vi "Create Debug Tool.vi"() -> (3 "array":T1)   [LabVIEW 2025, in "MCP Server.lvlib"]
uses:
  MCP Server.lvlib
  Tool Data.ctl
  Input Parameter.ctl
  Output Parameter.ctl
  Test_Tool.vi
  <vilib>/Utility/Data Type/NI_Data Type.lvlib
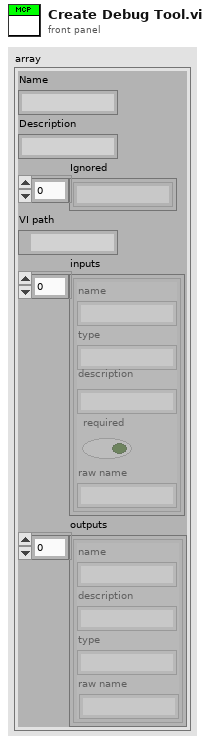
[diagram p1: front panel]
types:
  T1 = typedef "MCP Server.lvlib/Tool Data.ctl" = cluster{"Name":string, "Description":string, "Ignored":string[], "VI path":path, "inputs":T2[], "outputs":T3[]}
  T2 = typedef "MCP Server.lvlib/Input Parameter.ctl" = cluster{"name":string, "type":string, "description":string, "required":bool, "raw name":string}
  T3 = typedef "MCP Server.lvlib/Output Parameter.ctl" = cluster{"name":string, "description":string, "type":string, "raw name":string}
  T4 = enum16{"Invalid Wire Rule", "Required", "Recommended", "Optional", "Dynamic Dispatch"}[]
  T5 = enum16{"Invalid Wire Rule", "Required", "Recommended", "Optional", "Dynamic Dispatch"}
  T6 = typedef "NI_Data Type.lvlib/Data Type.ctl" = enum8{"Invalid Type", "Void", "I8", "I16", "I32", "I64", "U8", "U16", "U32", "U64", "Single Float", "Double Float", "Extended Float", "Single Complex", "Double Complex", "Extended Complex", "Enum U8", "Enum U16", "Enum U32", "Enum U64", "Single Float With Unit", "Double Float With Unit", "Extended Float With Unit", "Single Complex with Unit", "Double Complex with Unit", "Extended Complex with Unit", "Boolean", "String", "Path", "Picture", "Tag", "Array", "Cluster", "Variant", "LV Variant", "Waveform", "Timestamp", "Digital Waveform", "Digital Data", "ExpressData", "Refnum", "External Data", "VI", "Poly VI", "LabVIEW Class Instance", "Fixed Point", "Set Collection", "Map Collection"}
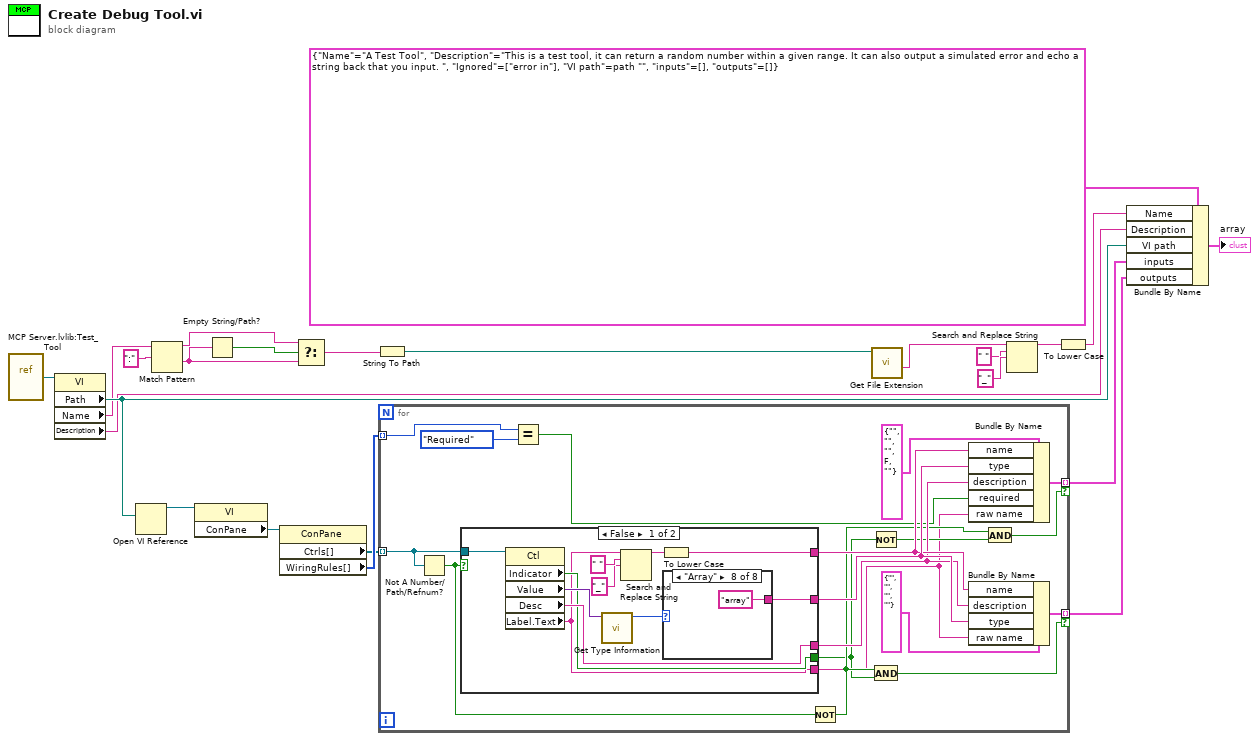
[diagram p0: block diagram]
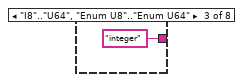
[diagram p4: hidden frame]
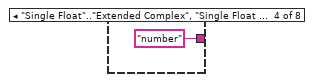
[diagram p5: hidden frame]
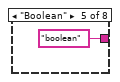
[diagram p6: hidden frame]
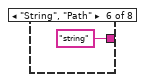
[diagram p7: hidden frame]
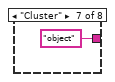
[diagram p8: hidden frame]
diagram:
  n1 = vi-ref "MCP Server.lvlib:Test_Tool.vi"() -> (w16:refnum<vi>)
  n2 = property class="VI"(reference=w16) -> ("Path"=w19:path, "Name"=w13:string, "Description"=w6:string)  [unwired: 1 in, 2 out]
  n3 = Open VI Reference(vi path=w19) -> (vi reference=w17:refnum<vi>)  [unwired: 5 in, 1 out]
  n4 = Match Pattern(string=w13, regular expression=":") -> (before substring=w10:string, after substring=w9:string)  [unwired: 1 in, 2 out]
  n5 = property class="VI"(reference=w17) -> ("ConPane"=w18:refnum<vi>)  [unwired: 1 in, 2 out]
  n6 = Empty String/Path?(string/path=w9) -> (empty?=w11:bool)
  n7 = property class="ConPane"(reference=w18) -> ("Ctrls[]"=w20:refnum<vi>[], "WiringRules[]"=w21:T4)  [unwired: 1 in, 2 out]
  n8 = Select(t=w10, s=w11, f=w9) -> (s? t:f=w8:string)
  n9 = String To Path(string=w8) -> (path=w7:path)
  n10 = for {
    tunnel: w20 -> [w39] mode=indexing
    tunnel: w21 -> [w28] mode=indexing
    tunnel: [w40] -> w22 mode=indexing if=w32
    tunnel: [w34] -> w23 mode=indexing if=w33
    n11 = Not A Number/Path/Refnum?(number/path/refnum=w39) -> (NaN/Path/Refnum?=w25:bool)
    n12 = case shown="False" w25 {
      tunnel: w39 -> [w52 _]
      tunnel: [w43 _] -> w36
      tunnel: [w51 _] -> w37
      tunnel: [w48 _] -> w35
      tunnel: [w47 _] -> w30
      tunnel: [w42 _] -> w24
      frame False {
        n13 = property class="Ctl"(reference=w52) -> ("Indicator"=w47:bool, "Value"=w50:variant, "Desc"=w48:string, "Label.Text"=w42:string)  [unwired: 1 in, 2 out]
        n14 = call <vilib>:"Get Type Information.vi"("variant"=w50) -> ("type"=w49:T6)  [unwired: 6 in, 4 out]
        n15 = Search and Replace String(input string=w42, search string=" ", replace string="_" ("replace string (\"\")")) -> (result string=w46:string)  [unwired: 5 in, 3 out]
        n16 = To Lower Case(string=w46) -> (all lower case string=w43:string)
        n17 = case shown="\"Array\"" w49 {
          tunnel: [_ _ "integer" ("JSON to Insert") "number" ("JSON to Insert") "boolean" ("JSON to Insert") "string" ("JSON to Insert") "object" ("JSON to Insert") "array" ("JSON to Insert")] -> w51
          frame "Invalid Type", Default {
          }
          frame "Void" {
          }
          frame "I8".."U64", "Enum U8".."Enum U64" {
          }
          frame "Single Float".."Extended Complex", "Single Float With Unit".."Extended Complex with Unit" {
          }
          frame "Boolean" {
          }
          frame "String", "Path" {
          }
          frame "Cluster" {
          }
          frame "Array" {
          }
        }
      }
      frame True {
      }
    }
    n18 = Equal?(x=w28, y=T5."Required") -> (x = y?=w26:bool)
    n19 = Not(x=w25) -> (.not. x?=w31:bool)
    n20 = Not(x=w30) -> (.not. x?=w29:bool)
    n21 = And(x=w31, y=w30) -> (x .and. y?=w33:bool)
    n22 = Bundle By Name(cluster=T2 {"name"="", "type"="", "description"="", "required"=FALSE, "raw name"=""} ("Cluster"), "name"=w36, "type"=w37, "description"=w35, "required"=w26, "raw name"=w24) -> (w40:T2)
    n23 = Bundle By Name(cluster=T3 {"name"="", "description"="", "type"="", "raw name"=""} ("outputs"), "name"=w36, "description"=w35, "type"=w37, "raw name"=w24) -> (w34:T3)
    n24 = And(x=w31, y=w29) -> (x .and. y?=w32:bool)
  }
  n25 = call <vilib>:"Get File Extension.vi"("file"=w7) -> ("filename without extension"=w2:string)  [unwired: 6 in, 4 out]
  n26 = Search and Replace String(input string=w2, search string=" ", replace string="_" ("replace string (\"\")")) -> (result string=w3:string)  [unwired: 5 in, 3 out]
  n27 = To Lower Case(string=w3) -> (all lower case string=w1:string)
  n28 = Bundle By Name(cluster=T1 {"Name"="A Test Tool", "Description"="This is a test tool, it can return a random number within a given range. It can also output a simulated error and echo a string back that you input. ", "Ignored"=["error in"], "VI path"=path "", "inputs"=[], "outputs"=[]} ("array"), "Name"=w1, "Description"=w6, "VI path"=w19, "inputs"=w22, "outputs"=w23) -> (→"array":T1)
